vi "Untitled 1.vi"() -> ()   [LabVIEW 2016]
panel:
  out "Signals Added":string[](array[string])
  out "Signals Removed":string[](array[string])
  out "SysDef Signals":string[](array[string])
  out "DLL Signals":string[](array[string])
  out "Parameters Added":string[](array[string])
  out "Parameters Removed":string[](array[string])
  out "SysDef Parameters":string[](array[string])
  out "DLL Parameters":string[](array[string])
  out "Outports Added":string[](array[string])
  out "Outports Removed":string[](array[string])
  out "SysDef Outports":string[](array[string])
  out "DLL Outports":string[](array[string])
  out "Inports Added":string[](array[string])
  out "Inports Removed":string[](array[string])
  out "SysDef Inports":string[](array[string])
  out "DLL Inports":string[](array[string])
  out "Error (out)":errorcluster
  in  "Error (in)":errorcluster
  in  "System Definition Filepath (.nivssdf)":path
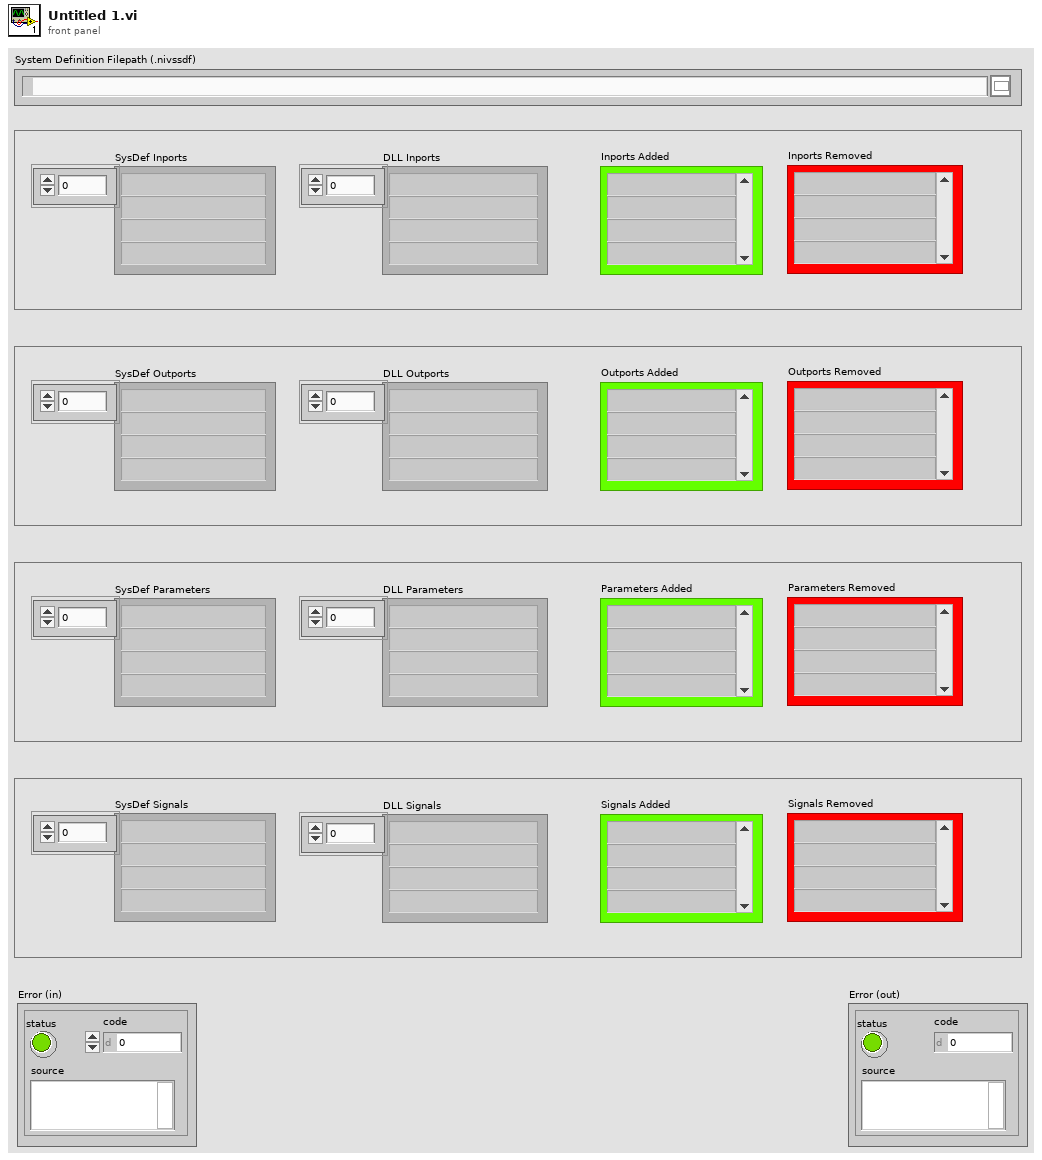
[diagram p1: front panel]
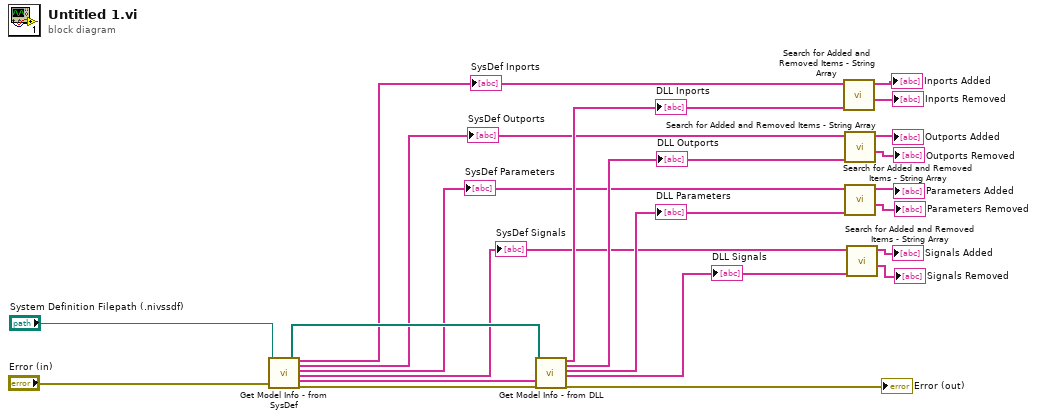
[diagram p0: block diagram]
diagram:
  n1 = call "Get Model Info - from SysDef.vi"("System Definition Filepath (.nivssdf)"="System Definition Filepath (.nivssdf)", "Error (in)"="Error (in)") -> ("Model Filepaths"=w18:path[], "SysDef Inports"=w15:string[], "SysDef Outports"=w10:string[], "SysDef Parameters"=w8:string[], "SysDef Signals"=w1:string[], "Models"=w17:string[], "Error (out)"=w20:errorcluster)  [unwired: 11 in]
  "SysDef Inports" <- w15
  "SysDef Outports" <- w10
  "SysDef Parameters" <- w8
  "SysDef Signals" <- w1
  n2 = call "Get Model Info - from DLL.vi"("Model Filepaths"=w18, "Models"=w17, "Error (in)"=w20) -> ("DLL Inports"=w16:string[], "DLL Outports"=w9:string[], "DLL Parameters"=w7:string[], "DLL Signals"=w2:string[], "Error (out)"=→"Error (out)":errorcluster)  [unwired: 12 in]
  "DLL Inports" <- w16
  "DLL Outports" <- w9
  "DLL Parameters" <- w7
  "DLL Signals" <- w2
  n3 = call "Search for Added and Removed Items - String Array.vi"("Model"=w16, "SysDef"=w15) -> ("Model Items Removed"=→"Inports Removed":string[], "Model Items Added"=→"Inports Added":string[])  [unwired: 8 in]
  n4 = call "Search for Added and Removed Items - String Array.vi"("Model"=w9, "SysDef"=w10) -> ("Model Items Removed"=→"Outports Removed":string[], "Model Items Added"=→"Outports Added":string[])  [unwired: 8 in]
  n5 = call "Search for Added and Removed Items - String Array.vi"("Model"=w7, "SysDef"=w8) -> ("Model Items Removed"=→"Parameters Removed":string[], "Model Items Added"=→"Parameters Added":string[])  [unwired: 8 in]
  n6 = call "Search for Added and Removed Items - String Array.vi"("Model"=w2, "SysDef"=w1) -> ("Model Items Removed"=→"Signals Removed":string[], "Model Items Added"=→"Signals Added":string[])  [unwired: 8 in]
